vi "Grow.vi"(8 "error in (no error)":errorcluster, 10 "Coordinates":T1, 11 "Snake in":refnum<class "Snake.lvclass">) -> (0 "error out":errorcluster, 3 "Snake out":refnum<class "Snake.lvclass">)   [LabVIEW 2018, in "Snake.lvclass"]
uses:
  Snake.lvclass
  Type Defs/Coordinates.ctl
  Snake.lvclass/Snake.ctl
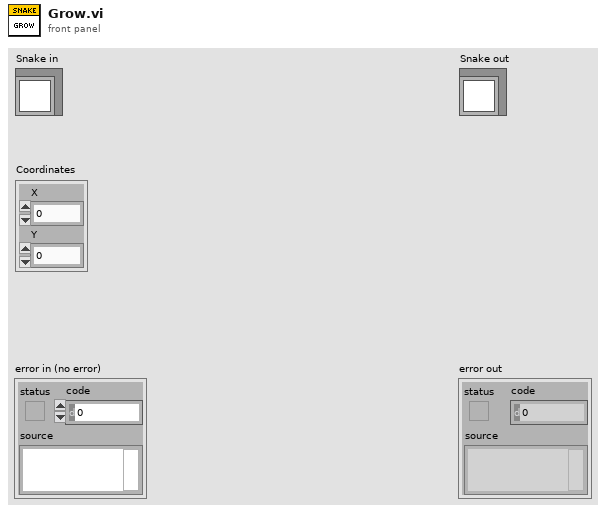
[diagram p1: front panel]
types:
  T1 = typedef "Coordinates.ctl" = cluster{"X":i32, "Y":i32}
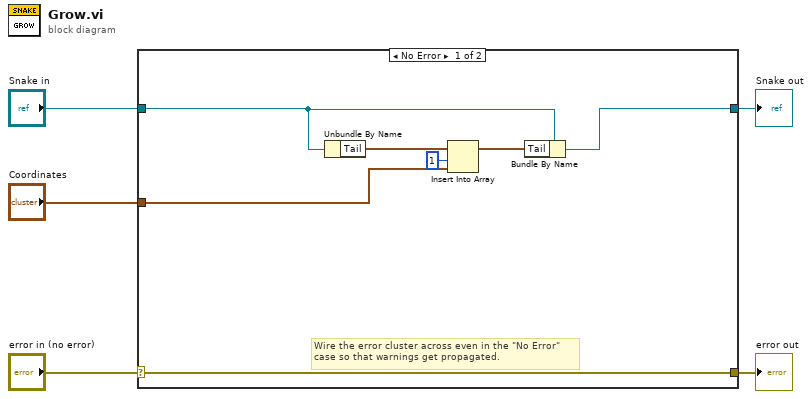
[diagram p0: block diagram]
diagram:
  n1 = case shown="No Error" "error in (no error)" {
    selector: "error in (no error)" -> [w12 w14]
    tunnel: [w12 w14] -> w4
    tunnel: [w10 w13] -> w2
    tunnel: "Snake in" -> [w11 w13]
    tunnel: "Coordinates" -> [w7 _]
    frame No Error {
      # "Wire the error cluster across even in the \"No Error\"\ncase so that warnings get propagated."
      n2 = Unbundle By Name(w11) -> ("Tail"=w9:T1[])
      n3 = Insert Into Array(array=w9, index=1, new element=w7) -> (w8:T1[])
      n4 = Bundle By Name(cluster=w11, "Tail"=w8) -> (w10:refnum<class "Snake.lvclass">)
    }
    frame Error {
    }
  }
  "error out" <- w4
  "Snake out" <- w2
